vi "Configure Frequency Domain.vi"(0 "VISA resource name":refnum<visa-resource-name>, 1 "FFT Window (0: fftBlackmanHarris)":i32(ring) items=["fftBlackmanHarris", "fftHann", "fftHamming", "fftEquiripple", "fftFlattop", "fftGaussian", "fftKaiser", "fftUniform", "fftRifeVincent4", "fftRifeVincent5", "fftRifeVincent10", "fftBlackmanHarris7"], 2 "Frequency Phase Unwrap (T: Enable)":bool=TRUE, 5 "Analyzer (0: A0)":i32(ring) items=["A0", "A1"], 7 "FFT Frequency Lines (0: fftl32k)":i32(ring) items=["fftl32k", "fftl16k", "fftl8k", "fftl4k", "fftl2k", "fftl1k", "fftl512", "fftl256"], 9 "Frequency Range (0: fftFsDiv2)":i32(ring) items=["fftFsDiv2", "fftFsDiv4", "fftFsDiv8", "fftFsDiv16", "fftFsDiv32", "fftFsDiv64", "fftFsDiv128", "fftFsDiv256", "fftFsDiv512", "fftFsDiv1024"], 11 "error in (no error)":errorcluster, 12 "Frequency Phase Threshold (0 dBUI)":dbl, 13 "Frequency DC Correction (0: jdcNone)":i32(ring) items=["jdcNone", "jdcAvg", "jdcHalfPkPk"]) -> (4 "VISA resource name out":refnum<visa-resource-name>, 15 "error out":errorcluster)   [LabVIEW 2014, in "Stanford Research SR1.lvlib"]
doc: "Configures the attributes for the Frequency Domain."
uses:
  Stanford Research SR1.lvlib
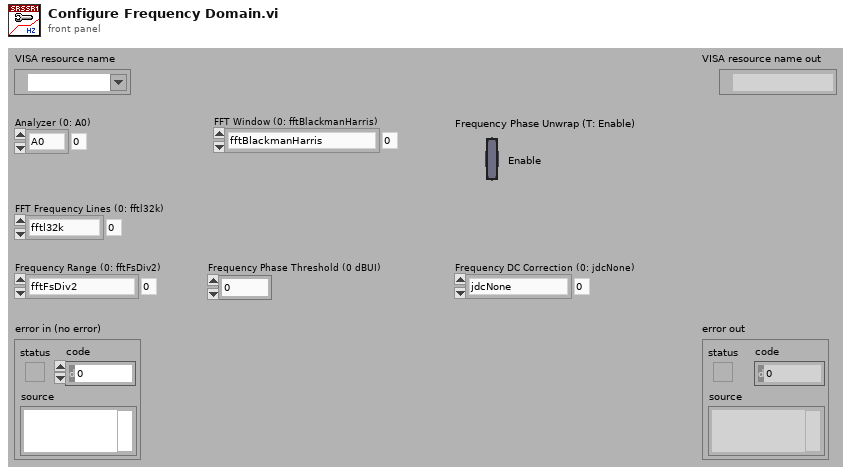
[diagram p1: front panel]
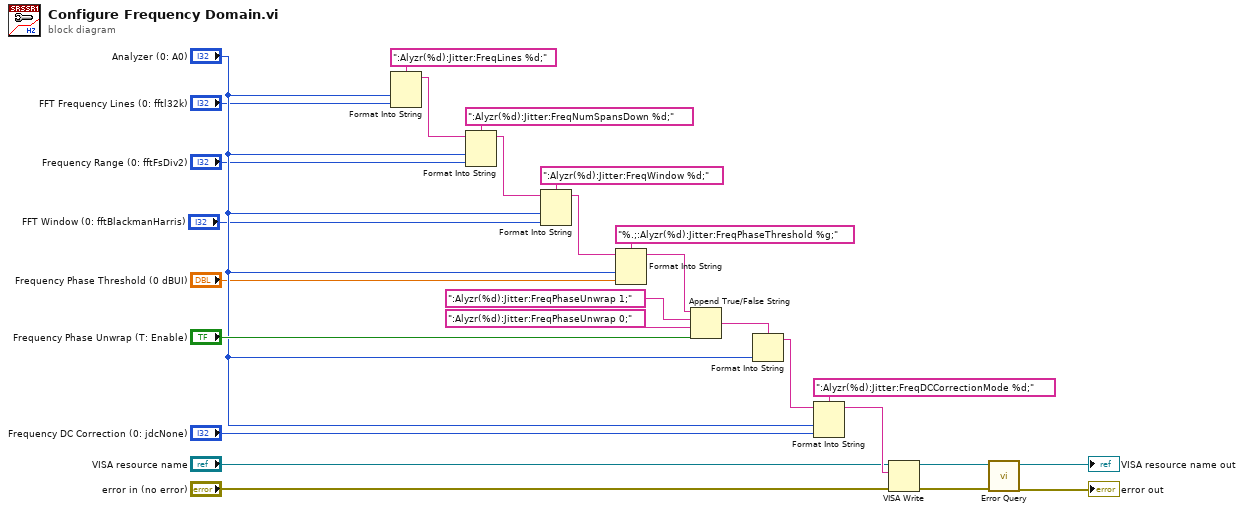
[diagram p0: block diagram]
diagram:
  n1 = Format Into String(format string=":Alyzr(%d):Jitter:FreqLines %d;", "Analyzer (0: A0)", "FFT Frequency Lines (0: fftl32k)") -> (resulting string=w26:string)  [unwired: 2 in, 1 out]
  n2 = Format Into String(format string=":Alyzr(%d):Jitter:FreqNumSpansDown %d;", initial string=w26, "Analyzer (0: A0)", "Frequency Range (0: fftFsDiv2)") -> (resulting string=w24:string)  [unwired: 1 in, 1 out]
  n3 = Format Into String(format string=":Alyzr(%d):Jitter:FreqWindow %d;", initial string=w24, "Analyzer (0: A0)", "FFT Window (0: fftBlackmanHarris)") -> (resulting string=w22:string)  [unwired: 1 in, 1 out]
  n4 = Format Into String(format string="%.;:Alyzr(%d):Jitter:FreqPhaseThreshold %g;", initial string=w22, "Analyzer (0: A0)", "Frequency Phase Threshold (0 dBUI)") -> (resulting string=w20:string)  [unwired: 1 in, 1 out]
  n5 = Append True/False String(1:"Frequency Phase Unwrap (T: Enable)", 2:":Alyzr(%d):Jitter:FreqPhaseUnwrap 0;", 3:":Alyzr(%d):Jitter:FreqPhaseUnwrap 1;", 4:w20) -> (0:w8:string)
  n6 = Format Into String(format string=w8, "Analyzer (0: A0)") -> (resulting string=w7:string)  [unwired: 2 in, 1 out]
  n7 = Format Into String(format string=":Alyzr(%d):Jitter:FreqDCCorrectionMode %d;", initial string=w7, "Analyzer (0: A0)", "Frequency DC Correction (0: jdcNone)") -> (resulting string=w15:string)  [unwired: 1 in, 1 out]
  n8 = VISA Write(VISA resource name="VISA resource name", write buffer=w15, error in (no error)="error in (no error)") -> (VISA resource name out=w12:refnum<visa-resource-name>, error out=w11:errorcluster)  [unwired: 1 out]
  n9 = call "Error Query.vi"("error in (no error)"=w11, "VISA resource name"=w12) -> ("error out"=→"error out":errorcluster, "VISA resource name out"=→"VISA resource name out":refnum<visa-resource-name>)  [unwired: 6 in, 2 out]
